vi "Set Values On Instances.vi"(8 "error in (no error)":errorcluster, 10 "Operations":T2(array[cluster]), 11 "Array":T1(array[cluster])) -> (0 "error out":errorcluster, 3 "output array":T1(array[cluster]))   [LabVIEW 2012]
uses:
  ClassDefinitions/SimpleClassWithMethods/SimpleArithmetic.lvclass
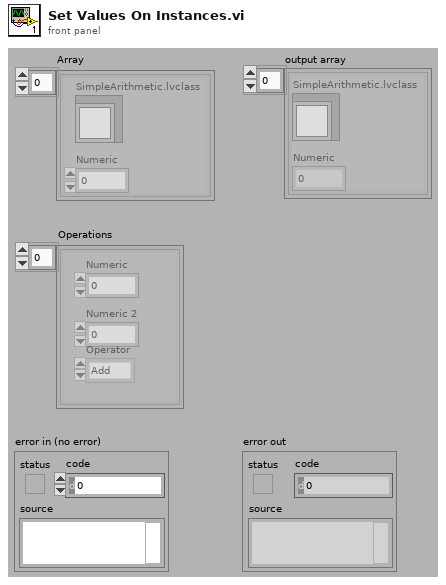
[diagram p1: front panel]
types:
  T1 = cluster{"SimpleArithmetic.lvclass":refnum<class "SimpleArithmetic.lvclass">, "Numeric":dbl}[]
  T2 = cluster{"Numeric":dbl, "Numeric 2":dbl, "Operator":enum16{"Add", "Divide", "Multiple", "Subtract"}}[]
  T3 = cluster{"SimpleArithmetic.lvclass":refnum<class "SimpleArithmetic.lvclass">, "Numeric":dbl}
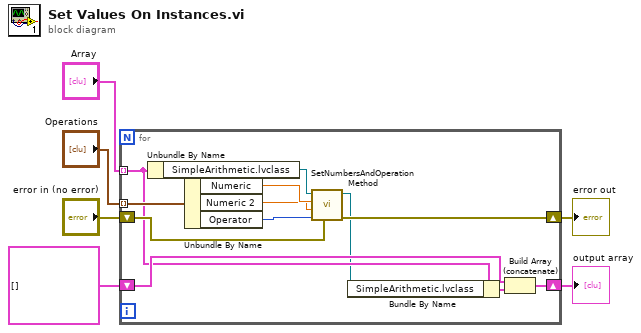
[diagram p0: block diagram]
diagram:
  n1 = for {
    tunnel: "Array" -> [w9] mode=indexing
    tunnel: "Operations" -> [w18] mode=indexing
    shift-right: [w11] -> w2
    shift-left: T1 [] ("Array") -> [w13]
    shift-right: [w12] -> w4
    shift-left: "error in (no error)" -> [w14]
    n2 = Unbundle By Name(w9) -> ("SimpleArithmetic.lvclass"=w10:refnum<class "SimpleArithmetic.lvclass">)
    n3 = Unbundle By Name(w18) -> ("Numeric"=w17:dbl, "Numeric 2"=w16:dbl, "Operator"=w15:enum16{"Add", "Divide", "Multiple", "Subtract"})
    n4 = call "SetNumbersAndOperationMethod.vi"("error in (no error)"=w14, "Operator"=w15, "Numeric 2"=w16, "Numeric"=w17, "SimpleArithmetic in"=w10) -> ("error out"=w12:errorcluster, "SimpleArithmetic out"=w7:refnum<class "SimpleArithmetic.lvclass">)  [unwired: 5 in]
    n5 = Bundle By Name(cluster=w9, "SimpleArithmetic.lvclass"=w7) -> (w8:T3)
    n6 = Build Array (concatenate)(w13, w8) -> (w11:T1)
  }
  "error out" <- w4
  "output array" <- w2
